vi "Test.vi"() -> ()   [LabVIEW 2015]
doc: "This VI is called when test mode begins, and will automatically be terminated when it ends. You can add manual or automatic tests and invoke them from the dashboard."
uses:
  <vilib>/functionblocks/Counter/Timer On Delay/Timer On Delay.vi
  <vilib>/functionblocks/FB Core/FB Core.xnode
  <vilib>/functionblocks/NI_FunctionBlock Libraries.lvlib
panel:
  out "Arm Difference (PID Input)":dbl
  out "Arm Angle":dbl
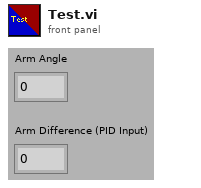
[diagram p1: front panel]
types:
  T1 = typedef "WPI_DigitalInputDevRef.ctl" = cluster{"DevStatus":errorcluster, "DIO Channel":T2}
  T2 = typedef "FPGA_DIOChannel.ctl" = enum8{"DIO 0", "DIO 1", "DIO 2", "DIO 3", "DIO 4", "DIO 5", "DIO 6", "DIO 7", "DIO 8", "DIO 9", "DIO MXP 0", "DIO MXP 1", "DIO MXP 2", "DIO MXP 3", "DIO MXP 4", "DIO MXP 5", "DIO MXP 6", "DIO MXP 7", "DIO MXP 8", "DIO MXP 9", "DIO MXP 10", "DIO MXP 11", "DIO MXP 12", "DIO MXP 13", "DIO MXP 14", "DIO MXP 15", "Invalid"}
  T3 = typedef "WPI_PotentiometerDevRef.ctl" = cluster{"DevStatus":errorcluster, "Analog Channel":T4, "Invert Output":bool}
  T4 = typedef "FPGA_AIChannel.ctl" = enum8{"AI 0", "AI 1", "AI 2", "AI 3", "AI MXP 0", "AI MXP 1", "AI MXP 2", "AI MXP 3", "Invalid"}
  T5 = cluster{bool, "output":bool, bool, bool, bool, bool, bool, dbl}
  T6 = typedef "WPI_ServoDeviceRef.ctl" = cluster{"DeviceStatus":errorcluster, "PWM Channel":T7, "DeadBand":T8}
  T7 = typedef "FPGA_DIOPWMChannel.ctl" = enum8{"PWM 0", "PWM 1", "PWM 2", "PWM 3", "PWM 4", "PWM 5", "PWM 6", "PWM 7", "PWM 8", "PWM 9", "PWM MXP 0", "PWM MXP 1", "PWM MXP 2", "PWM MXP 3", "PWM MXP 4", "PWM MXP 5", "PWM MXP 6", "PWM MXP 7", "PWM MXP 8", "PWM MXP 9", "Invalid"}
  T8 = typedef "WPI_PWMDeadband.ctl" = cluster{"Name":string, "maxPositivePwm":i32, "minPositivePwm":i32, "centerPwm":i32, "maxNegativePwm":i32, "minNegativePwm":i32, "angularRange":u16}
  T9 = cluster{"Arm Angle":dbl, "Angle Difference (PID Ref)":dbl}
  T10 = cluster{string, string, string, string, string, string, string, string}
  T11 = cluster{bool, bool, bool, bool, bool, bool, bool, bool}
  T12 = typedef "WPI_MotorControlDeviceRef.ctl" = cluster{"DeviceStatus":errorcluster, "Type":T13, "PWM":cluster{"PWM Channel":T7, "DeadBand":T8}, "CAN":cluster{"Device Number":u8, "Control Mode":T14, "Semaphore":T15, "Max Vout":dbl, "TalonSRX Control Mode":T16}, "Invert":bool}
  T13 = typedef "WPI_MotorControlType.ctl" = enum16{"PWM", "CAN", "CANTalonSRX"}
  T14 = typedef "WPI_CANJaguar_ControlMode.ctl" = enum8{"Percent VBus", "Current", "Speed", "Position", "Voltage"}
  T15 = typedef "Semaphore RefNum" = refnum<k1>
  T16 = typedef "WPI_CANTalonSRX_APIControlMode.ctl" = enum8{"Percent VBus", "Speed", "Position", "Slave", "Unchanged / Invalid", "Voltage Compensation", "Current", "Motion Profile"}
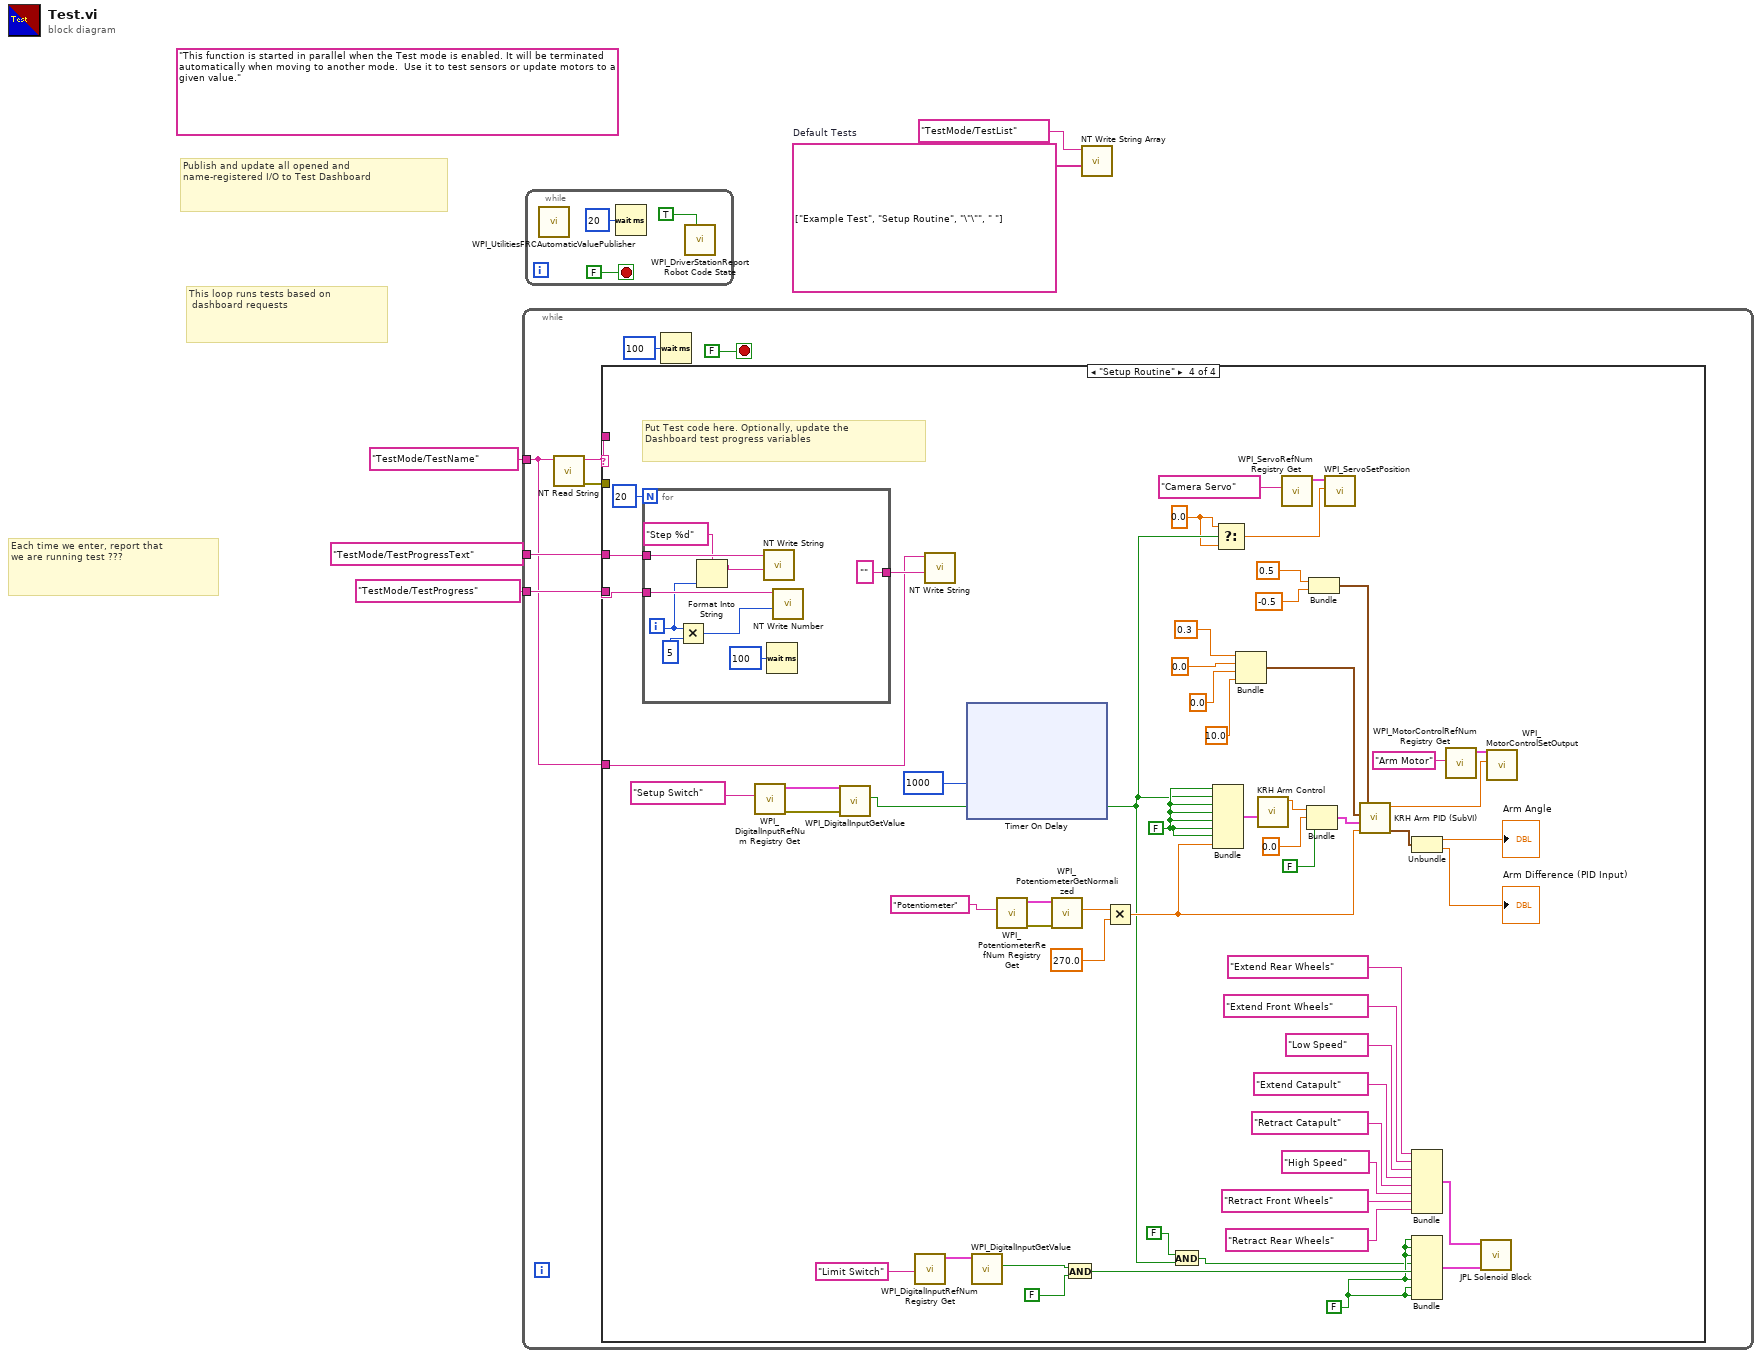
[diagram p0: block diagram]
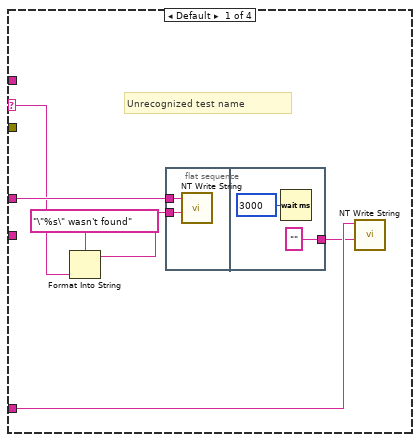
[diagram p2: hidden frame]
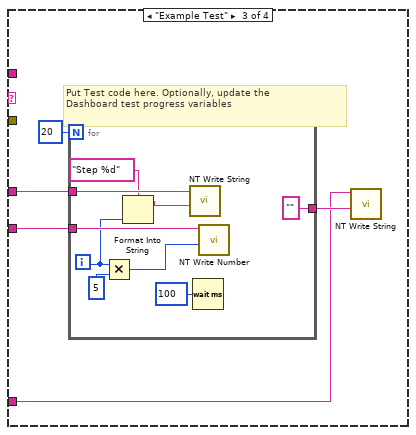
[diagram p4: hidden frame]
diagram:
  w2 = string[] ["Example Test", "Setup Routine", "\"\"", " "]  # Default Tests
  (unwired) "This function is started in parallel when the Test mode is enabled. It will be terminated automatically when moving to another mode.  Use it to test sensors or update motors to a given value."
  # "This loop runs tests based on \n dashboard requests"
  # "Publish and update all opened and\nname-registered I/O to Test Dashboard"
  # "Each time we enter, report that\nwe are running test ???"
  n1 = while {
    tunnel: "TestMode/TestName" ("Name") -> [w7]
    tunnel: "TestMode/TestProgressText" ("Name") -> [w10]
    tunnel: "TestMode/TestProgress" ("Name") -> [w9]
    stop <- FALSE stop-if-true
    n2 = call <vilib>:"NT Read String.vi"("Name"=w7) -> ("error out"=w6:errorcluster, "String"=w8:string)  [unwired: 9 in]
    n3 = case shown="\"Setup Routine\"" w8 {
      selector: w8 -> [w17 _ _ _]
      tunnel: w7 -> [w14 _ w23 w93]
      tunnel: w10 -> [w18 _ w26 w91]
      tunnel: w9 -> [_ _ w27 w92]
      tunnel: w8 -> [_ _ _ _]
      tunnel: w6 -> [_ _ _ _]
      frame Default {
        # "Unrecognized test name"
        n4 = Format Into String(format string="\"%s\" wasn't found" ("Name"), w17) -> (resulting string=w16:string)  [unwired: 2 in, 1 out]
        n5 = flat-sequence {
          tunnel: w18 -> [w19]
          tunnel: w16 -> [w20]
          tunnel: ["" ("Name")] -> w13
          frame #0 {
            n6 = call <vilib>:"NT Write String.vi"("String"=w20, "Name"=w19) -> ()  [unwired: 9 in, 1 out]
          }
          frame #1 {
            n7 = Wait (ms)(milliseconds to wait=u32 3000) -> ()  [unwired: 1 out]
          }
        }
        n8 = call <vilib>:"NT Write String.vi"("String"=w13, "Name"=w14) -> ()  [unwired: 9 in, 1 out]
      }
      frame "" {
        # "No test to run"
      }
      frame "Example Test" {
        # "Put Test code here. Optionally, update the\nDashboard test progress variables"
        n9 = for {
          N: 20 -> [_]
          tunnel: w27 -> [w36]
          tunnel: w26 -> [w34]
          tunnel: ["" ("String")] -> w24
          i -> [w31]
          n10 = Multiply(x=w31, y=u32 5 ("milliseconds to wait")) -> (x*y=w32:u32)
          n11 = Format Into String(format string="Step %d", w31) -> (resulting string=w29:string)  [unwired: 2 in, 1 out]
          n12 = call <vilib>:"NT Write String.vi"("String"=w29, "Name"=w34) -> ()  [unwired: 9 in, 1 out]
          n13 = Wait (ms)(milliseconds to wait=u32 100) -> ()  [unwired: 1 out]
          n14 = call <vilib>:"NT Write Number.vi"("Numeric"=w32, "Name"=w36) -> ()  [unwired: 9 in, 1 out]
        }
        n15 = call <vilib>:"NT Write String.vi"("String"=w24, "Name"=w23) -> ()  [unwired: 9 in, 1 out]
      }
      frame "Setup Routine" {
        w37 = 0.0
        w70 = FALSE
        w89 = FALSE
        # "Put Test code here. Optionally, update the\nDashboard test progress variables"
        n16 = for {
          N: 20 -> [_]
          tunnel: w92 -> [w146]
          tunnel: w91 -> [w144]
          tunnel: ["" ("String")] -> w94
          i -> [w141]
          n17 = Multiply(x=w141, y=u32 5 ("milliseconds to wait")) -> (x*y=w142:u32)
          n18 = Format Into String(format string="Step %d", w141) -> (resulting string=w139:string)  [unwired: 2 in, 1 out]
          n19 = call <vilib>:"NT Write String.vi"("String"=w139, "Name"=w144) -> ()  [unwired: 9 in, 1 out]
          n20 = Wait (ms)(milliseconds to wait=u32 100) -> ()  [unwired: 1 out]
          n21 = call <vilib>:"NT Write Number.vi"("Numeric"=w142, "Name"=w146) -> ()  [unwired: 9 in, 1 out]
        }
        n22 = call <vilib>:"WPI_DigitalInputRefNum Registry Get.vi"("refnum name"="Setup Switch") -> ("error out"=w59:errorcluster, "DigitalInputDevRef"=w60:T1)  [unwired: 9 in]
        n23 = call <vilib>:"WPI_DigitalInputGetValue.vi"("error in (no error)"=w59, "DigitalInputDevRef"=w60) -> ("Value"=w45:bool)  [unwired: 7 in, 2 out]
        n24 = call <vilib>:"WPI_DigitalInputRefNum Registry Get.vi"("refnum name"="Limit Switch") -> ("DigitalInputDevRef"=w72:T1)  [unwired: 9 in, 1 out]
        n25 = call <vilib>:"NT Write String.vi"("String"=w94, "Name"=w93) -> ()  [unwired: 9 in, 1 out]
        n26 = xnode "Timer On Delay"("preset time (ms)"=1000, "input"=w45) -> ("output"=w38:bool)  [unwired: 1 in, 2 out]
        n27 = call <vilib>:"WPI_DigitalInputGetValue.vi"("DigitalInputDevRef"=w72) -> ("Value"=w73:bool)  [unwired: 8 in, 2 out]
        n28 = call <vilib>:"WPI_PotentiometerRefNum Registry Get.vi"("refnum name"="Potentiometer") -> ("error out"=w83:errorcluster, "PotDevRef"=w84:T3)  [unwired: 9 in]
        n29 = call <vilib>:"WPI_PotentiometerGetNormalized.vi"("error in"=w83, "PotDevRef"=w84) -> ("Normalized Value"=w85:dbl)  [unwired: 7 in, 2 out]
        n30 = And(x=w73, y=FALSE) -> (x .and. y?=w74:bool)
        n31 = Multiply(x=w85, y=270.0) -> (x*y=w88:dbl)
        n32 = And(x=FALSE, y=w38) -> (x .and. y?=w43:bool)
        n33 = Bundle(w89, "output"=w38, w89, w89, w89, w89, w89, w88) -> (w87:T5)  [unwired: 1 in]
        n34 = Select(t=w37, s=w38, f=w37) -> (s? t:f=w39:dbl)
        n35 = Bundle(0.3, 0.0, 0.0, 10.0) -> (w80:cluster{dbl, dbl, dbl, dbl})  [unwired: 1 in]
        n36 = call "KRH Arm Control.vi"("Button Control"=w87) -> ("Arm Angle"=w46:dbl)  [unwired: 10 in]
        n37 = call <vilib>:"WPI_ServoRefNum Registry Get.vi"("refnum name"="Camera Servo") -> ("ServoDeviceRef"=w41:T6)  [unwired: 9 in, 1 out]
        n38 = Bundle("Arm Angle"=w46, 0.0, FALSE) -> (w79:cluster{"Arm Angle":dbl, dbl, bool})  [unwired: 1 in]
        n39 = Bundle(0.5, -0.5) -> (w81:cluster{dbl, dbl})  [unwired: 1 in]
        n40 = call <vilib>:"WPI_ServoSetPosition.vi"("Position"=w39, "ServoDeviceRef"=w41) -> ()  [unwired: 8 in, 2 out]
        n41 = call "KRH Arm PID (SubVI).vi"("Actual Angle"=w88, "Arm Control"=w79, "PID Settings"=w80, "PID Limits"=w81) -> ("Arm Status"=w77:T9, "output"=w78:dbl)  [unwired: 2 in]
        n42 = Unbundle(w77) -> ("Arm Angle"=→"Arm Angle":dbl, "Angle Difference (PID Ref)"=→"Arm Difference (PID Input)":dbl)
        n43 = Bundle("Extend Rear Wheels", "Extend Front Wheels", "Low Speed", "Extend Catapult", "Retract Catapult", "High Speed", "Retract Front Wheels", "Retract Rear Wheels") -> (w75:T10)  [unwired: 1 in]
        n44 = Bundle(w70, w70, w70, w43, w74, w70, w70, w70) -> (w76:T11)  [unwired: 1 in]
        n45 = call <vilib>:"WPI_MotorControlRefNum Registry Get.vi"("refnum name"="Arm Motor") -> ("MotorControlDevRef"=w56:T12)  [unwired: 9 in, 1 out]
        n46 = call "JPL Solenoid Block.vi"("Boolean Inputs"=w76, "References"=w75) -> ()  [unwired: 9 in, 1 out]
        n47 = call <vilib>:"WPI_MotorControlSetOutput.vi"("Output"=w78, "MotorControlDevRef"=w56) -> ()  [unwired: 7 in, 3 out]
      }
    }
    n48 = Wait (ms)(milliseconds to wait=u32 100) -> ()  [unwired: 1 out]
  }
  n49 = while {
    stop <- FALSE stop-if-true
    n50 = call <vilib>:"WPI_UtilitiesFRCAutomaticValuePublisher.vi"() -> ()  [unwired: 12 in]
    n51 = Wait (ms)(milliseconds to wait=u32 20) -> ()  [unwired: 1 out]
    n52 = call <vilib>:"WPI_DriverStationReport Robot Code State.vi"("Test"=TRUE ("Autonomous")) -> ()  [unwired: 10 in, 1 out]
  }
  n53 = call <vilib>:"NT Write String Array.vi"("String Array"=w2, "Name"="TestMode/TestList") -> ()  [unwired: 9 in, 1 out]
